vi "IO_DataQ_Measure.vi"() -> ()   [LabVIEW 2024]
doc: "This example performs writes and reads on a serial port, as directed by the user. You can press the Write and Read buttons, and change the Read Count, while the example is running.\n\nThe parameters set for the serial port must match the parameters of the connected instrument or device. In this example, the Read Count parameter specifies the number of bytes that the serial port reads. If there were more bytes at the port than the specified number, those bytes would not be read. If there were less bytes at the port than the specified number, you would receive a timeout error.\n\nThis example expands upon the flow control options for XON and XOFF, allowing the user to choose those control characters. Also, the user can enable or disable a termination character. Some devices require a termination character in order to identify the end of command strings. Some devices send a termination character to signify the end of data to be read. This example shows how you can end the Read operation once a termination character is detected in the buffer and/or append a termination character at the end of the Write data."
uses:
  <vilib>/Instr/_visa.llb/VISA Configure Serial Port (Instr).vi
panel:
  out "AI Outs":dbl[](array[numeric])
  in  "Command List":string="srate 6000\nps 2\ndec 100\ndeca 1\nnop\n"
  out "Read Buf":string[](array[string])
  in  "Filter":bool=TRUE
  out "Packet Count":u32=20
  in  "Num Packets":u32=20
  out "Sample Rate":dbl=98.82643607164917
  out "Num Bytes":u32=1280
  out "Meas Loop Time":u32=6476
  out "x/y":dbl=218.425
  out "millisecond timer value 4":u32=833776
  out "millisecond timer value 3":u32=615351
  out "Total Time":u32=218425
  out "Loop time":u32[](array[numeric])=[0, 5, 5, 5, 5, 5, 5, 5, 5, 6, 4, 5, 5, 6, 4, 5, 5, 5, 6, 4, 5, 5, 5, 5, 5, 5, 5, 5, 5, 5, 5, 6, 4, 6, 5, 5, 4, 5, 5, 6, 4, 5, 5, 5, 6, 4, 5, 6, 4, 5, 5, 5, 5, 5, 5, 6, 4, 5, 5, 5, 5, 5, 5, 5, 5, 7, 3, 5, 5, 5, 5, 5, 5, 5, 5, 5, 6, 5, 4, 6, 4, 5, 5, 5, 6, 4, 5, 5, 5, 5, 6, 6, 4, 4, 5, 5, 6, 4, 5, 5, 5, 6, 6, 3, 5, 5, 6, 4, 5, 5, 5, 5, 5, 5, 5, 5, 5, 5, 5, 5, 5, 6, 5, 4, 6, 5, 5, 5, 4, 5, 5, 6, 4, 5, 5, 6, 4, 5, 6, 4, 6, 4, 5, 6, 4, 6, 5, 4, 6, 4, 5, 6, 4, 5, 6, 4, 6, 4, 5, 5, 5, 5, 5, 5, 5, 5, 5, 6, 4, 5, 5, 5, 5, 6, 4, 5, 5, 5, 5, 5, 5, 5, 5, 5, 5, 7, 3, 5, 5, 6, 4, 5, 6, 5, 4, 5, 5, 5, 5, 6, 5, 4, 5, 5, 5, 5, 5, 8, 2, 6, 6, 3, 5, 5, 6, 5, 4, 5, 5, 6, 5, 4, 5, 5, 5, 5, 5, 6, 4, 5, 5, 6, 4, 5, 5, 5, 5, 5, 5, 5, 5, 5, 5, 5, 6, 4, 5, 5, 5, 5, 5, 5, 5, 6, 4, 5, 6, 4, 5, 5, 5, 6, 5, 4, 5, 5, 5, 6, 4, 5, 5, 5, 5, 5, 5, 5, 5, 5, 6, 4, 5, 6, 4, 5, 6, 4, 5, 5, 5, 5, 5, 5, 5, 5, 5, 5, 6, 4, 5, 6, 4, 6, 4, 6, 4, 5, 5, 5, 5, 5, 6, 5, 5, 4, 5, 5, 6, 4, 5, 5, 5, 5, 5, 6, 5, 5, 5, 4, 5, 5, 5, 5, 6, 4, 5, 5, 5, 5, 6, 5, 4, 6, 4, 5, 5, 5, 5, 5, 5, 6, 4, 5, 5, 5, 6, 5, 4, 5, 5, 5, 5, 5, 5, 5, 6, 5, 5, 4, 6, 5, 5, 4, 5, 6, 4, 5, 5, 5, 5, 5, 5, 5, 5, 5, 5, 5, 6, 4, 5, 6, 5, 4, 6, 4, 6, 4, 5, 5, 5, 5, 6, 4, 6, 4, 5, 5, 5, 6, 4, 5, 6, 5, 4, 5, 5, 5, 7, 3, 5, 5, 5, 5, 5, 5, 6, 4, 6, 4, 5, 6, 4, 5, 5, 5, 5, 5, 5, 5, 5, 5, 5, 5, 5, 5, 5, 5, 5, 5, 5, 5, 6, 4, 5, 5, 5, 5, 5, 6, 4, 5, 6, 4, 5, 5, 5, 5, 6, 4, 5, 5, 5, 6, 4, 5, 5, 5, 6, 4, 5, 6, 4, 5, 6, 4, 7, 3, 5, 5, 5, 6, 4, 6, 4, 6, 5, 4, 5, 5, 5, 6, 5, 4, 5, 5, 5, 5, 5, 5, 5, 5, 5, 5, 5, 5, 5, 5, 5, 5, 5, 5, 5, 5, 6, 4, 5, 5, 6, 4, 5, 6, 4, 5, 5, 5, 5, 6, 4, 6, 4, 5, 5, 5, 5, 5, 5, 5, 6, 4, 5, 5, 5, 5, 5, 6, 5, 4, 6, 4, 5, 5, 5, 5, 5, 5, 5, 6, 5, 4, 6, 5, 4, 6, 4, 5, 6, 4, 5, 5, 6, 5, 5, 4, 6, 5, 4, 5, 6, 4, 5, 5, 5, 5, 5, 5, 5, 5, 5, 5, 5, 6, 4, 5, 6, 5, 4, 5, 6, 5, 5, 4, 6, 5, 4, 5, 6, 4, 5, 5, 5, 5, 5, 5, 6, 4, 5, 5, 6, 4, 5, 5, 5, 5, 5, 6, 4, 5, 5, 5, 5, 5, 5, 6, 4, 5, 5, 5, 5, 5, 5, 6, 4, 5, 6, 4, 5, 5, 5, 5, 6, 4, 5, 5, 5, 6, 4, 5, 5, 5, 6, 4, 5, 5, 5, 5, 5, 5, 5, 5, 5, 5, 5, 5, 6, 5, 5, 5, 4, 5, 5, 5, 5, 5, 5, 5, 5, 5, 5, 5, 5, 5, 5, 6, 5, 4, 5, 5, 6, 6, 3, 6, 4, 5, 6, 4, 5, 5, 6, 4, 5, 6, 4, 5, 6, 4, 5, 6, 5, 4, 5, 5, 5, 5, 5, 5, 5, 6, 4, 6, 4, 5, 6, 4, 5, 5, 5, 5, 5, 5, 5, 5, 5, 5, 5, 5, 5, 6, 5, 4, 5, 6, 5, 4, 6, 4, 5, 5, 5, 5, 5, 6, 4, 5, 6, 4, 7, 3, 5, 5, 5, 5, 5, 5, 5, 5, 5, 5, 6, 4, 5, 5, 5, 5, 5, 6, 5, 5, 4, 5, 5, 5, 6, 4, 6, 5, 5, 4, 5, 5, 5, 5, 7, 4, 4, 5, 5, 5, 5, 5, 5, 6, 5, 4, 5, 5, 6, 4, 5, 5, 5, 5, 5, 5, 5, 5, 5, 5, 5, 5, 5, 5, 5, 5, 6, 5, 4, 6, 4, 5, 6, 4, 5, 5, 6, 5, 4, 6, 4, 5, 5, 6, 4, 5, 6, 4, 6, 4, 5, 6, 4, 5, 5, 5, 6, 4, 5, 6, 4, 6, 4, 6, 4, 5, 5, 5, 5, 5, 5, 5, 5, 5, 5, 5, 5, 5, 5, 5, 5, 5, 5, 5, 5, 6, 4, 5, 6, 4, 5, 6, 4, 5, 6, 4, 5, 5, 5, 5, 5, 5, 6, 4, 5, 5, 5, 5, 5, 5, 5, 5, 5, 6, 4, 5, 5, 5, 5, 5, 5, 5, 5, 6, 4, 5, 5, 5, 5, 5, 5, 5, 5, 5, 5, 6, 5, 4, 5, 5, 5, 5, 6, 5, 4, 5, 5, 5, 5, 6, 4, 5, 6, 4, 5, 5, 5, 5, 5, 5, 5, 5, 5, 5, 5, 5, 5, 5, 5, 5, 5, 5, 5, 5, 5, 6, 4, 5, 5, 6, 4, 5, 5, 5, 5, 5, 6, 4, 5, 5, 6, 5, 4, 5, 6, 4, 5, 5, 5, 5, 5, 5, 5, 5, 7, 3, 5, 5, 5, 5, 5, 5, 6, 4, 5, 5, 5, 5, 5, 5, 5, 5, 5, 5, 5, 5, 5, 5, 5, 5, 5, 6, 4, 5, 6, 4, 5, 5, 5, 5, 7, 3, 6, 4, 5, 5, 6, 4, 5, 5, 5, 6, 4, 5, 5, 6, 6, 3, 5, 5, 5, 5, 5, 5, 5, 5, 5, 5, 5, 5, 5, 5, 5, 5, 5, 5, 5, 5, 5, 5, 5, 5, 5, 5, 5, 5, 5, 5, 5, 5, 5, 5, 6, 4, 5, 5, 6, 4, 6, 4, 5, 5, 5, 7, 3, 5, 6, 4, 5, 6, 4, 5, 5, 5, 5, 5, 5, 5, 5, 5, 6, 4, 5, 5, 5, 5, 6, 4, 5, 5, 5, 5, 6, 5, 4, 5, 5, 5, 5, 5, 5, 5, 5, 5, 6, 4, 6, 5, 4, 5, 5, 6, 4, 5, 5, 5, 6, 4, 5, 5, 5, 5, 5, 5, 5, 6, 4, 5, 5, 5, 5, 5, 6, 4, 5, 6, 5, 5, 4, 5, 5, 6, 4, 5, 5, 5, 6, 5, 5, 4, 5, 6, 4, 7, 4, 5, 5, 4, 5, 5, 5, 5, 6, 4, 5, 5, 5, 6, 5, 4, 5, 5, 5, 5, 5, 5, 5, 5, 5, 5, 6, 5, 4, 5, 5, 5, 5, 7, 4, 4, 6, 4, 6, 5, 4, 5, 5, 5, 5, 5, 6, 5, 4, 5, 6, 5, 4, 6, 4, 5, 5, 5, 5, 5, 5, 5, 5, 5, 5, 5, 5, 5, 5, 5, 5, 6, 4, 5, 6, 4, 5, 6, 4, 5, 5, 5, 6, 4, 6, 5]
  out "millisecond timer value 2":u32=833776
  out "millisecond timer value":u32=827300
  in  "Num Chan":i32=1
  out "Loop Time":i32=6475
  out "Array":u32[](array[numeric])=[0, 0, 0, 0, 0, 0, 64, 64, 64, 128, 128, 128, 128, 192, 192, 192, 192, 256, 256, 256, 320, 320, 320, 384, 384, 384, 384, 384, 448, 448, 448, 448, 512, 512, 576, 576, 576, 576, 640, 640, 640, 704, 704, 704, 768, 768, 768, 832, 832, 832, 896, 896, 896, 896, 960, 960, 960, 960, 1024, 1024, 1024, 1088, 1088, 1088, 1088, 1152, 1152, 1152, 1152, 1152, 1216, 1216, 1216, 1280, 1280, 1280, 1280, 1344, 1344, 1344, 1344, 1408, 1408, 1408, 1472, 1472, 1472, 1536, 1536, 1536, 1600, 1600, 1600, 1600, 1664, 1664, 1664, 1664, 1728, 1728]
  out "size(s)":i32[](array[numeric])=[0, 0, 0, 0, 0, 0, 0, 0, 0, 0, 0, 0, 0, 0, 0, 0, 0, 0, 0, 0, 0, 0, 0, 0, 0, 0, 0, 0, 0, 0, 0, 0, 0, 0, 0, 0, 0, 0, 0, 0, 0, 0, 0, 0, 0, 0, 0, 0, 0, 0, 0, 0, 0, 0, 0, 0, 0, 0, 0, 0, 0, 0, 0, 0, 0, 0, 0, 0, 0, 0, 0, 0, 0, 0, 0, 0, 0, 0, 0, 64, 0, 0, 0, 0, 0, 0, 0, 0, 0, 0, 0, 0, 0, 0, 0, 0, 0, 0, 0, 0, 0, 0, 0, 0, 0, 0, 0, 0, 0, 0, 0, 0, 0, 0, 0, 0, 0, 0, 0, 0, 0, 0, 0, 0, 0, 0, 0, 0, 0, 0, 0, 0, 0, 0, 0, 0, 0, 0, 0, 0, 0, 0, 0, 64, 0, 0, 0, 0, 0, 0, 0, 0, 0, 0, 0, 0, 0, 0, 0, 0, 0, 0, 0, 0, 0, 0, 0, 0, 0, 0, 0, 0, 0, 0, 0, 0, 0, 0, 0, 0, 0, 0, 0, 0, 0, 0, 0, 0, 0, 0, 0, 0, 0, 0, 0, 0, 0, 0, 0, 0, 0, 0, 0, 0, 0, 0, 0, 64, 0, 0, 0, 0, 0, 0, 0, 0, 0, 0, 0, 0, 0, 0, 0, 0, 0, 0, 0, 0, 0, 0, 0, 0, 0, 0, 0, 0, 0, 0, 0, 0, 0, 0, 0, 0, 0, 0, 0, 0, 0, 0, 0, 0, 0, 0, 0, 0, 0, 0, 0, 0, 0, 0, 0, 0, 0, 0, 0, 0, 0, 0, 0, 64, 0, 0, 0, 0, 0, 0, 0, 0, 0, 0, 0, 0, 0, 0, 0, 0, 0, 0, 0, 0, 0, 0, 0, 0, 0, 0, 0, 0, 0, 0, 0, 0, 0, 0, 0, 0, 0, 0, 0, 0, 0, 0, 0, 0, 0, 0, 0, 0, 0, 0, 0, 0, 0, 0, 0, 0, 0, 0, 0, 0, 0, 0, 0, 64, 0, 0, 0, 0, 0, 0, 0, 0, 0, 0, 0, 0, 0, 0, 0, 0, 0, 0, 0, 0, 0, 0, 0, 0, 0, 0, 0, 0, 0, 0, 0, 0, 0, 0, 0, 0, 0, 0, 0, 0, 0, 0, 0, 0, 0, 0, 0, 0, 0, 0, 0, 0, 0, 0, 0, 0, 0, 0, 0, 0, 0, 0, 0, 64, 0, 0, 0, 0, 0, 0, 0, 0, 0, 0, 0, 0, 0, 0, 0, 0, 0, 0, 0, 0, 0, 0, 0, 0, 0, 0, 0, 0, 0, 0, 0, 0, 0, 0, 0, 0, 0, 0, 0, 0, 0, 0, 0, 0, 0, 0, 0, 0, 0, 0, 0, 0, 0, 0, 0, 0, 0, 0, 0, 0, 0, 0, 0, 64, 0, 0, 0, 0, 0, 0, 0, 0, 0, 0, 0, 0, 0, 0, 0, 0, 0, 0, 0, 0, 0, 0, 0, 0, 0, 0, 0, 0, 0, 0, 0, 0, 0, 0, 0, 0, 0, 0, 0, 0, 0, 0, 0, 0, 0, 0, 0, 0, 0, 0, 0, 0, 0, 0, 0, 0, 0, 0, 0, 0, 0, 0, 64, 0, 0, 0, 0, 0, 0, 0, 0, 0, 0, 0, 0, 0, 0, 0, 0, 0, 0, 0, 0, 0, 0, 0, 0, 0, 0, 0, 0, 0, 0, 0, 0, 0, 0, 0, 0, 0, 0, 0, 0, 0, 0, 0, 0, 0, 0, 0, 0, 0, 0, 0, 0, 0, 0, 0, 0, 0, 0, 0, 0, 0, 0, 0, 0, 64, 0, 0, 0, 0, 0, 0, 0, 0, 0, 0, 0, 0, 0, 0, 0, 0, 0, 0, 0, 0, 0, 0, 0, 0, 0, 0, 0, 0, 0, 0, 0, 0, 0, 0, 0, 0, 0, 0, 0, 0, 0, 0, 0, 0, 0, 0, 0, 0, 0, 0, 0, 0, 0, 0, 0, 0, 0, 0, 0, 0, 0, 0, 0, 64, 0, 0, 0, 0, 0, 0, 0, 0, 0, 0, 0, 0, 0, 0, 0, 0, 0, 0, 0, 0, 0, 0, 0, 0, 0, 0, 0, 0, 0, 0, 0, 0, 0, 0, 0, 0, 0, 0, 0, 0, 0, 0, 0, 0, 0, 0, 0, 0, 0, 0, 0, 0, 0, 0, 0, 0, 0, 0, 0, 0, 0, 0, 0, 64, 0, 0, 0, 0, 0, 0, 0, 0, 0, 0, 0, 0, 0, 0, 0, 0, 0, 0, 0, 0, 0, 0, 0, 0, 0, 0, 0, 0, 0, 0, 0, 0, 0, 0, 0, 0, 0, 0, 0, 0, 0, 0, 0, 0, 0, 0, 0, 0, 0, 0, 0, 0, 0, 0, 0, 0, 0, 0, 0, 0, 0, 0, 0, 64, 0, 0, 0, 0, 0, 0, 0, 0, 0, 0, 0, 0, 0, 0, 0, 0, 0, 0, 0, 0, 0, 0, 0, 0, 0, 0, 0, 0, 0, 0, 0, 0, 0, 0, 0, 0, 0, 0, 0, 0, 0, 0, 0, 0, 0, 0, 0, 0, 0, 0, 0, 0, 0, 0, 0, 0, 0, 0, 0, 0, 0, 0, 0, 64, 0, 0, 0, 0, 0, 0, 0, 0, 0, 0, 0, 0, 0, 0, 0, 0, 0, 0, 0, 0, 0, 0, 0, 0, 0, 0, 0, 0, 0, 0, 0, 0, 0, 0, 0, 0, 0, 0, 0, 0, 0, 0, 0, 0, 0, 0, 0, 0, 0, 0, 0, 0, 0, 0, 0, 0, 0, 0, 0, 0, 0, 0, 0, 64, 0, 0, 0, 0, 0, 0, 0, 0, 0, 0, 0, 0, 0, 0, 0, 0, 0, 0, 0, 0, 0, 0, 0, 0, 0, 0, 0, 0, 0, 0, 0, 0, 0, 0, 0, 0, 0, 0, 0, 0, 0, 0, 0, 0, 0, 0, 0, 0, 0, 0, 0, 0, 0, 0, 0, 0, 0, 0, 0, 0, 0, 0, 0, 64, 0, 0, 0, 0, 0, 0, 0, 0, 0, 0, 0, 0, 0, 0, 0, 0, 0, 0, 0, 0, 0, 0, 0, 0, 0, 0, 0, 0, 0, 0, 0, 0, 0, 0, 0, 0, 0, 0, 0, 0, 0, 0, 0, 0, 0, 0, 0, 0, 0, 0, 0, 0, 0, 0, 0, 0, 0, 0, 0, 0, 0, 0, 0, 64, 0, 0, 0, 0, 0, 0, 0, 0, 0, 0, 0, 0, 0, 0, 0, 0, 0, 0, 0, 0, 0, 0, 0, 0, 0, 0, 0, 0, 0, 0, 0, 0, 0, 0, 0, 0, 0, 0, 0, 0, 0, 0, 0, 0, 0, 0, 0, 0, 0, 0, 0, 0, 0, 0, 0, 0, 0, 0, 0, 0, 0, 0, 0, 64, 0, 0, 0, 0, 0, 0, 0, 0, 0, 0, 0, 0, 0, 0, 0, 0, 0, 0, 0, 0, 0, 0, 0, 0, 0, 0, 0, 0, 0, 0, 0, 0, 0, 0, 0, 0, 0, 0, 0, 0, 0, 0, 0, 0, 0, 0, 0, 0, 0, 0, 0, 0, 0, 0, 0, 0, 0, 0, 0, 0, 0, 0, 0, 64, 0, 0, 0, 0, 0, 0, 0, 0, 0, 0, 0, 0, 0, 0, 0, 0, 0, 0, 0, 0, 0, 0, 0, 0, 0, 0, 0, 0, 0, 0, 0, 0, 0, 0, 0, 0, 0, 0, 0, 0, 0, 0, 0, 0, 0, 0, 0, 0, 0, 0, 0, 0, 0, 0, 0, 0, 0, 0, 0, 0, 0, 0, 0, 64, 0, 0, 0, 0, 0, 0, 0, 0, 0, 0, 0, 0, 0, 0, 0, 0, 0, 0, 0, 0, 0, 0, 0, 0, 0, 0, 0, 0, 0, 0, 0, 0, 0, 0, 0, 0, 0, 0, 0, 0, 0, 0, 0, 0, 0, 0, 0, 0, 0, 0, 0, 0, 0, 0, 0, 0, 0, 0, 0, 0, 0, 0, 0, 64]
  out "Waveform Chart":dbl[][](graph)=[[3.57208251953125], [3.55621337890625], [3.55621337890625], [3.55621337890625], [3.56170654296875], [3.56689453125], [3.56170654296875], [3.56170654296875], [3.55621337890625], [3.56170654296875], [3.56170654296875], [3.55621337890625], [3.56689453125], [3.56170654296875], [3.55621337890625], [3.56170654296875], [3.56689453125], [3.56170654296875], [3.56170654296875], [3.56689453125], [3.56170654296875], [3.57208251953125], [3.56170654296875], [3.57208251953125], [3.56170654296875], [3.55621337890625], [3.55621337890625], [3.56689453125], [3.551025390625], [3.56170654296875], [3.55621337890625], [3.56170654296875]]
  in  "Stop":bool
  in  "2108 CDC Virtual COM":refnum<visa-resource-name>="COM3"
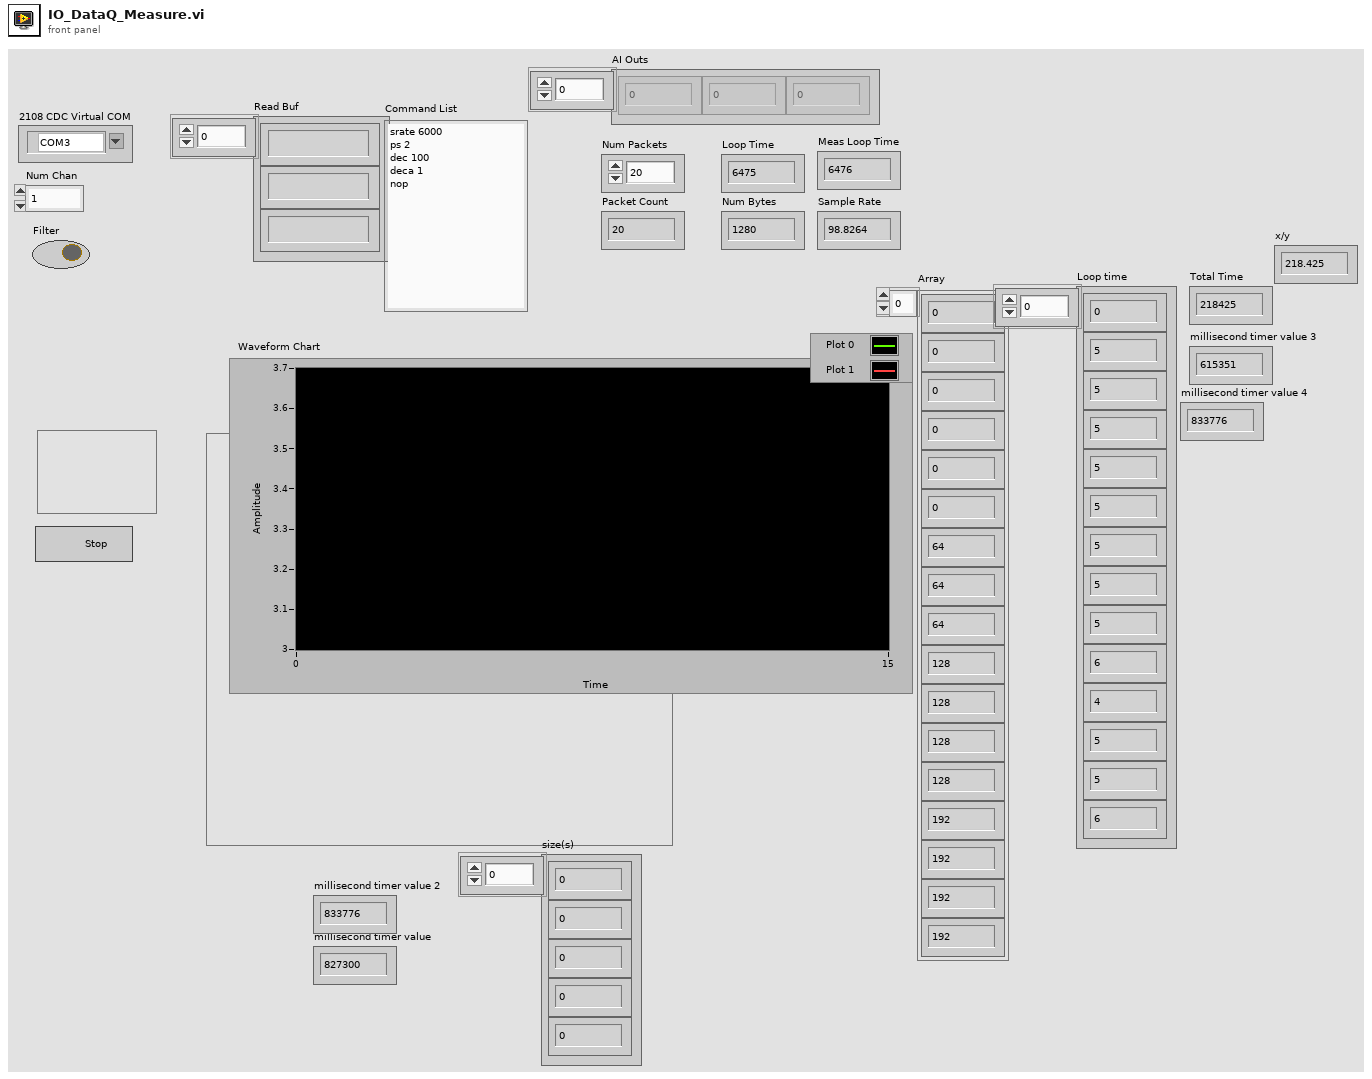
[diagram p1: front panel]
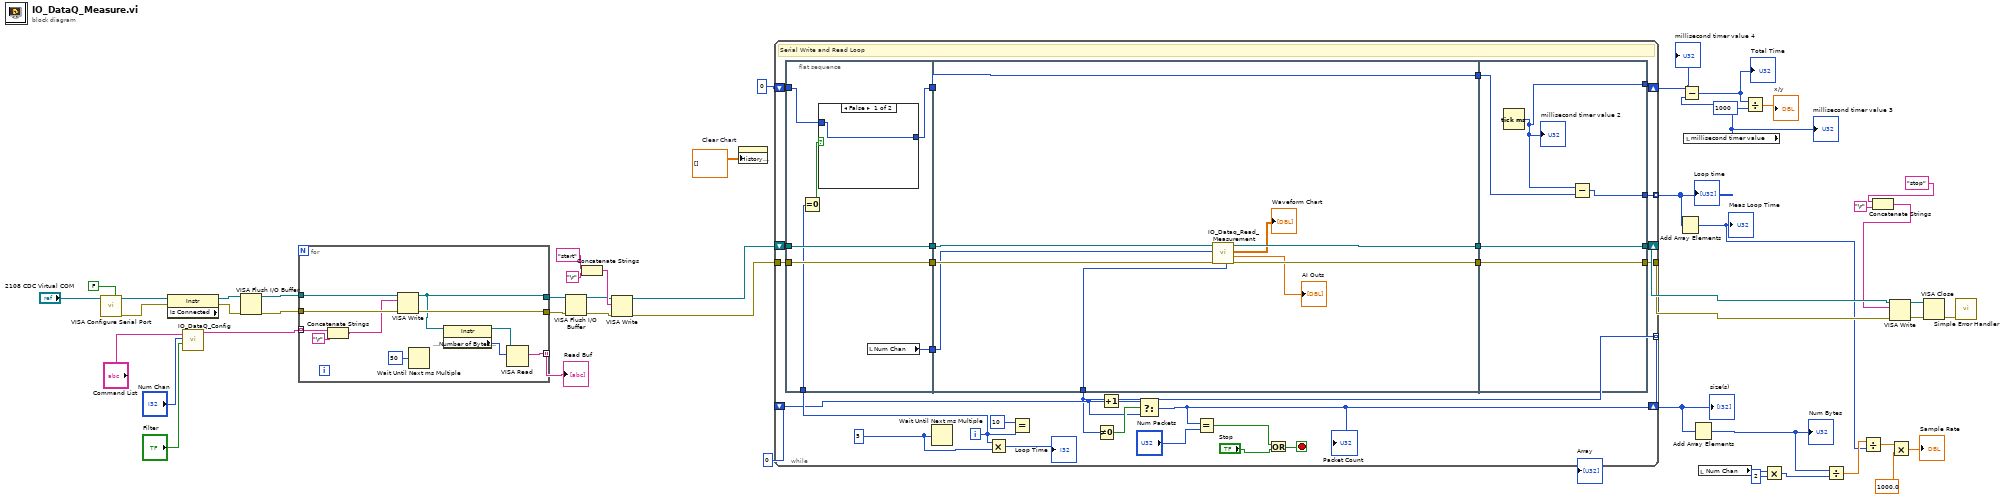
[diagram p0: block diagram]
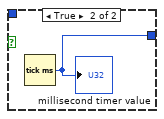
[diagram p2: hidden frame]
diagram:
  n1 = call-poly "VISA Configure Serial Port"("VISA resource name"="2108 CDC Virtual COM", "Enable Termination\nChar (T)"=FALSE) -> ("VISA resource name out"=w47:refnum<visa-resource-name>, "error out"=w49:errorcluster)  [unwired: 8 in, 4 out]
  n2 = property class="Instr" props=["Is Connected"](reference=w47, error in=w49) -> (reference out=w8:refnum<visa-resource-name>, error out=w7:errorcluster)  [unwired: 1 out]
  n3 = call "IO_DataQ_Config.vi"("Filter"="Filter", "Num Chan"="Num Chan", "Command List"="Command List") -> ("Array"=w4:string[])  [unwired: 8 in]
  n4 = VISA Flush I/O Buffer(VISA resource name=w8, error in (no error)=w7) -> (VISA resource name out=w6:refnum<visa-resource-name>, error out=w5:errorcluster)  [unwired: 1 in]
  n5 = for {
    tunnel: w4 -> [w58] mode=indexing
    tunnel: w6 -> [w60]
    tunnel: w5 -> [w59]
    tunnel: [w55] -> w32
    tunnel: [w57] -> w30
    tunnel: [w51] -> w9 mode=indexing
    n6 = Concatenate Strings(w58, "\r") -> (w52:string)
    n7 = VISA Write(VISA resource name=w60, write buffer=w52, error in (no error)=w59) -> (VISA resource name out=w55:refnum<visa-resource-name>, error out=w57:errorcluster)  [unwired: 1 out]
    n8 = Wait Until Next ms Multiple(millisecond multiple=u32 50) -> ()  [unwired: 1 out]
    n9 = property class="Instr"(reference=w55) -> (reference out=w53:refnum<visa-resource-name>, "Serial Settings:Number of Bytes at Serial Port"=w54:u32)  [unwired: 1 in, 1 out]
    n10 = VISA Read(VISA resource name=w53, byte count=w54) -> (read buffer=w51:string)  [unwired: 1 in, 3 out]
  }
  "Read Buf" <- w9
  n11 = VISA Flush I/O Buffer(VISA resource name=w32, error in (no error)=w30) -> (VISA resource name out=w31:refnum<visa-resource-name>, error out=w29:errorcluster)  [unwired: 1 in]
  n12 = Concatenate Strings("start", "\r") -> (w36:string)
  n13 = VISA Write(VISA resource name=w31, write buffer=w36, error in (no error)=w29) -> (VISA resource name out=w35:refnum<visa-resource-name>, error out=w34:errorcluster)  [unwired: 1 out]
  n14 = property on="Clear Chart" class="WFChart (strict)"("History Data"=dbl[][] []) -> ()  [unwired: 2 in, 2 out]
  n15 = while {
    shift-right: [w87] -> w45
    shift-left: w35 -> [w85]
    tunnel: w34 -> [w84]
    tunnel: [w86] -> w42
    tunnel: [w77] -> w21 mode=indexing
    shift-right: [w76] -> w27
    shift-left: u32 0 ("millisecond timer value") -> [w73]
    shift-right: [w62] -> _
    shift-left: u32 0 ("Bytes at Port") -> [w66]
    tunnel: [w63] -> w19 mode=indexing
    i -> [w71]
    stop <- w83 stop-if-true
    w70 = u32 5 ("milliseconds to wait")
    # "Serial Write and Read Loop"
    n16 = flat-sequence {
      tunnel: w84 -> [w93]
      tunnel: w85 -> [w94]
      tunnel: [w94] -> w81
      tunnel: [w93] -> w80
      tunnel: [w91] -> w74
      tunnel: w73 -> [w90]
      tunnel: w71 -> [w89]
      tunnel: [w88] -> w61
      tunnel: w81 -> [w103]
      tunnel: w80 -> [w101]
      tunnel: [w105] -> w79
      tunnel: [w104] -> w78
      tunnel: [w102] -> w75
      tunnel: w74 -> [w102]
      tunnel: [w97] -> w63
      tunnel: w61 -> [w100]
      tunnel: [w109] -> w86
      tunnel: [w110] -> w87
      tunnel: w79 -> [w110]
      tunnel: w78 -> [w109]
      tunnel: [w108] -> w77
      tunnel: [w107] -> w76
      tunnel: w75 -> [w106]
      frame #0 {
        n17 = Equal To 0?(x=w89) -> (x = 0?=w92:bool)
        n18 = case shown="False" w92 {
          tunnel: [w95 w96] -> w91
          tunnel: w90 -> [w95 _]
          frame False {
          }
          frame True {
            n19 = Tick Count (ms)() -> (millisecond timer value=w96:u32)
            "millisecond timer value" <- w96
          }
        }
        n20 = local read "Num Chan"() -> (w88:i32)
      }
      frame #1 {
        n21 = call "IO_Dataq_Read_Measurement.vi"("error in (no error)"=w101, "Num Chan"=w100, "VISA Refnum in"=w103) -> ("error out"=w104:errorcluster, "Outputs"=→"AI Outs":dbl[], "Waveform Chart"=→"Waveform Chart":dbl[][], "VISA Refnum out"=w105:refnum<visa-resource-name>, "Bytes at Port"=w97:u32)  [unwired: 4 in]
      }
      frame #2 {
        n22 = Tick Count (ms)() -> (millisecond timer value=w107:u32)
        "millisecond timer value 2" <- w107
        n23 = Subtract(x=w107, y=w106) -> (x-y=w108:u32)
      }
    }
    n24 = Wait Until Next ms Multiple(millisecond multiple=w70) -> ()  [unwired: 1 out]
    n25 = Multiply(x=w71, y=w70) -> (x*y=→"Loop Time":u32)
    n26 = Equal?(x=10, y=w71) -> ()  [unwired: 1 out]
    n27 = Not Equal To 0?(x=w63) -> (x != 0?=w68:bool)
    n28 = Increment(x=w66) -> (x+1=w67:u32)
    n29 = Select(t=w67, s=w68, f=w66) -> (s? t:f=w62:u32)
    "Packet Count" <- w62
    n30 = Equal?(x=w62, y="Num Packets") -> (x = y?=w64:bool)
    n31 = Or(x=w64, y="Stop") -> (x .or. y?=w83:bool)
  }
  "Loop time" <- w21
  "millisecond timer value 4" <- w27
  "size(s)" <- w19
  n32 = Add Array Elements(numeric array=w21) -> (sum=w10:u32)
  "Meas Loop Time" <- w10
  n33 = local read "millisecond timer value"() -> (w26:u32)
  "millisecond timer value 3" <- w26
  n34 = Subtract(x=w27, y=w26) -> (x-y=w25:u32)
  "Total Time" <- w25
  n35 = Add Array Elements(numeric array=w19) -> (sum=w15:u32)
  "Num Bytes" <- w15
  n36 = local read "Num Chan"() -> (w18:i32)
  n37 = Divide(x=w25, y=u32 1000) -> (x/y=→"x/y":dbl)
  n38 = Multiply(x=w18, y=2) -> (x*y=w16:i32)
  n39 = Divide(x=w15, y=w16) -> (x/y=w11:dbl)
  n40 = Divide(x=w11, y=w10) -> (x/y=w14:dbl)
  n41 = Concatenate Strings("stop", "\r") -> (w39:string)
  n42 = VISA Write(VISA resource name=w45, write buffer=w39, error in (no error)=w42) -> (VISA resource name out=w44:refnum<visa-resource-name>, error out=w43:errorcluster)  [unwired: 1 out]
  n43 = Multiply(x=w14, y=1000.0) -> (x*y=→"Sample Rate":dbl)
  n44 = VISA Close(VISA resource name=w44, error in (no error)=w43) -> (error out=w48:errorcluster)
  n45 = call <vilib>:"Simple Error Handler.vi"("error in (no error)"=w48) -> ()  [unwired: 1 in, 8 out]
